vi "PointScan Galvo.vi"(11 "Input Coords":dbl[](array[numeric])) -> (0 "AI out":refnum<k21>, 1 "AO out":refnum<k21>)   [LabVIEW 2020]
uses:
  <resource>/objmgr/daqmx.rc
  <vilib>/DAQmx/create/channels.llb/DAQmx Create Channel (AO-Voltage-Basic).vi
  <vilib>/DAQmx/create/channels.llb/DAQmx Create Channel (AI-Voltage-Basic).vi
  <vilib>/DAQmx/configure/timing.llb/DAQmx Timing (Sample Clock).vi
  <vilib>/DAQmx/write.llb/DAQmx Write (Analog 2D DBL NChan NSamp).vi
panel:
  out "array":dbl[][](array[numeric])
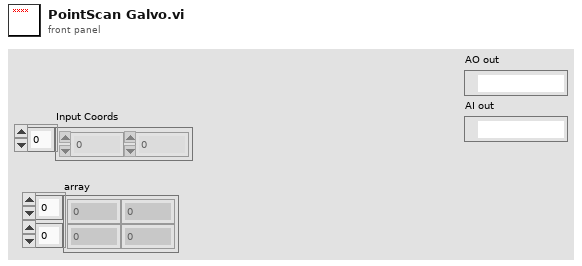
[diagram p1: front panel]
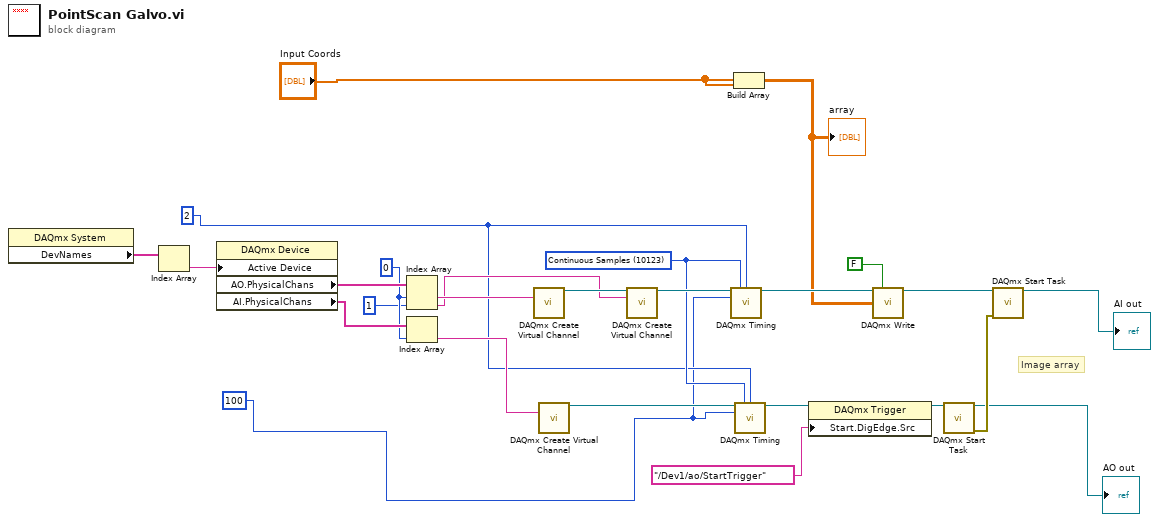
[diagram p0: block diagram]
diagram:
  w4 = 2
  w3 = 100
  w7 = 10123 items=["Finite Samples"=10178, "Continuous Samples"=10123, "Hardware Timed Single Point"=12522] ("sample mode")
  w22 = 0 ("index")
  # "Image array"
  n1 = property class="DAQmx System"() -> ("DevNames"=w26:tag[])  [unwired: 2 in, 2 out]
  n2 = Index Array(array=w26) -> (element=w25:tag)  [unwired: 1 in]
  n3 = property class="DAQmx Device"("Active Device"=w25) -> ("AO.PhysicalChans"=w24:tag[], "AI.PhysicalChans"=w23:tag[])  [unwired: 2 in, 2 out]
  n4 = Index Array(array=w24, index #1=w22, index #2=1 ("index")) -> (element #1=w20:tag, element #2=w18:tag)
  n5 = Index Array(array=w23, index=w22) -> (element=w17:tag)
  n6 = call-poly <vilib>:"DAQmx Create Virtual Channel.vi"("physical channels"=w20) -> ("task out"=w19:refnum<k21>)  [unwired: 13 in, 1 out]
  n7 = call-poly <vilib>:"DAQmx Create Virtual Channel.vi"("physical channels"=w17) -> ("task out"=w16:refnum<k21>)  [unwired: 13 in, 1 out]
  n8 = call-poly <vilib>:"DAQmx Create Virtual Channel.vi"("task in"=w19, "physical channels"=w18) -> ("task out"=w15:refnum<k21>)  [unwired: 12 in, 1 out]
  n9 = call-poly <vilib>:"DAQmx Timing.vi"("task/channels in"=w15, "sample mode"=w7, "samples per channel"=w4, "rate"=w3) -> ("task out"=w10:refnum<k21>)  [unwired: 10 in, 1 out]
  n10 = Build Array("Input Coords", "Input Coords") -> (w1:dbl[][])
  "array" <- w1
  n11 = call-poly <vilib>:"DAQmx Timing.vi"("task/channels in"=w16, "sample mode"=w7, "samples per channel"=w4, "rate"=w3) -> ("task out"=w14:refnum<k21>)  [unwired: 10 in, 1 out]
  n12 = property class="DAQmx Trigger"(reference=w14, "Start.DigEdge.Src"=tag "/Dev1/ao/StartTrigger") -> (reference out=w12:refnum<k21>)  [unwired: 1 in, 1 out]
  n13 = call-poly <vilib>:"DAQmx Write.vi"("task/channels in"=w10, "auto start"=FALSE, "data"=w1) -> ("task out"=w9:refnum<k21>)  [unwired: 10 in, 2 out]
  n14 = call <vilib>:"DAQmx Start Task.vi"("task/channels in"=w12) -> ("task out"=→"AO out":refnum<k21>, "error out"=w11:errorcluster)  [unwired: 13 in]
  n15 = call <vilib>:"DAQmx Start Task.vi"("task/channels in"=w9, "error in"=w11) -> ("task out"=→"AI out":refnum<k21>)  [unwired: 12 in, 1 out]
